vi "OverallControl.vi"(10 "Settings":T1={"Name of test"="", "Date"=timestamp(0 s since 1904-01-01), "Location"="", "Template"="", "Soundcard"="", "resolution"=0, "Sampling rate"=0, "Ch1 Gain "=0.0, "Ch2 Gain"=0.0, "Sample time (s)"=0.0, "Pre-trigger (s)"=0.0, "Hammer Threshold"=0.0, "Positions"=0, "Taps/Position"=0, "Set Names"="", "Freq resolution"=0.0, "Hammer cutoff"=0.0, "Mic cutoff"=0.0, "Double bounce "=0.0, "Hammer Cal"=0.0, "dB Offset"=0.0, "Accel Cal"=0.0, "Vibrometer Cal"=0.0, "Mic Cal"=0.0, "Output"=0, "Voltage Cal"=0.0, "Vibrometer Port"="", "Range"=0, "High Pass"=0, "Bandwidth"=0, "X Range"=[], "Y Range"=[], "dB Spread"=0.0, "Trigger"=0, "Ch_1"=0, "Ch_2"=0, "flip?"=FALSE, "60Hz"=FALSE, "Time offset"=0.0, "Piezo Cal"=1.0, "Default Notes"=""} {"Ch_2" min=1 step=1; "Ch_1" min=1 max=100 step=1; "Trigger" items=["Hammer (force)", "Self-tap", "Spacebar"]; "Bandwidth" items=["1 kHz"=1, "5 kHz"=5, "10 kHz"=10, "25 kHz"=25, "50 kHz"=50, "100 kHz"=100]; "High Pass" items=["Off", "13 Hz", "104 Hz"]; "Range" items=["10 mm/s"=1, "20 mm/s"=2, "50 mm/s"=5, "100 mm/s"=10, "200 mm/s"=20, "500 mm/s"=50, "1 m/s"=100, "2 m/s"=200]; "Output" items=["Accelerometer", "Speed (from acceleration)", "Microphone", "Vibrometer", "Piezo"]; "Voltage Cal" format="%#_13g"; "Ch2 Gain" format="%#_13g"; "Ch1 Gain" format="%#_13g"; "Double bounce" min=0.0; "Mic cutoff" min=0.0 format="%#_4g"; "Hammer cutoff" min=0.0 format="%#_4g"; "Freq resolution" min=0.0; "Pre-trigger (s)" format="%#_13g"; "Date" format="%<%H:%M\n%d/%m/%y>T"; "resolution" items=["16 bit"=16, "24 bit"=24, "32 bit"=32]; "Sampling rate" items=["22050 samp/s"=22050, "44100 samp/s"=44100, "48000 samp/s"=48000]}) -> (1 "Success?":bool, 3 "VISA Refnum out":refnum<visa-resource-name>)   [LabVIEW 2022 SP3]
uses:
  PreferencesControl.ctl
panel:
  out "Sent":string
  out "String Read":string
  # "Hz"
  # "dB"
  # "dB"
  # "sec"
  # "sec"
  # "mV/Pa"
  # "mV/m/s2"
  # "mV/mm/s"
  # "V/N"
  # "sec"
  # "sec"
  # "mV/N"
  # "a.u."
  # "a.u."
  # "sec"
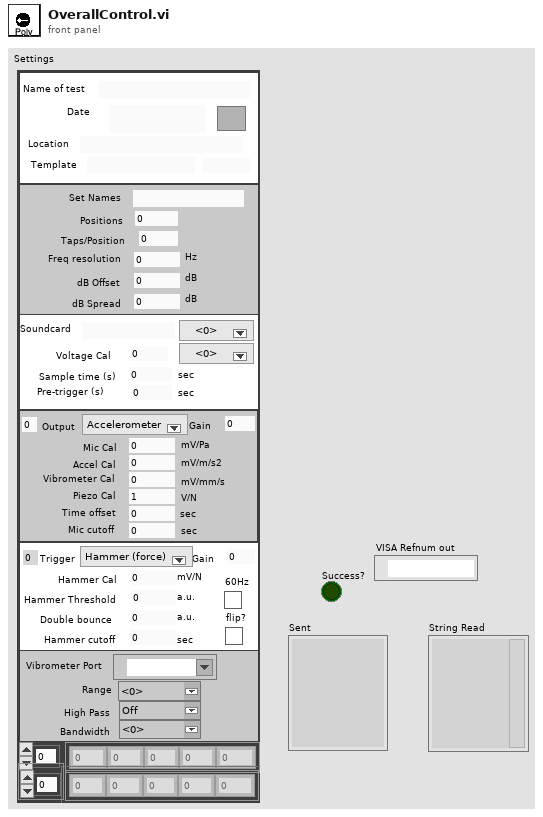
[diagram p1: front panel]
types:
  T1 = typedef "PreferencesControl.ctl" = cluster{"Name of test":string, "Date":timestamp, "Location":string, "Template":string, "Soundcard":string, "resolution":u16, "Sampling rate":u16, "Ch1 Gain ":dbl, "Ch2 Gain":dbl, "Sample time (s)":dbl, "Pre-trigger (s)":dbl, "Hammer Threshold":dbl, "Positions":i16, "Taps/Position":i16, "Set Names":string, "Freq resolution":dbl, "Hammer cutoff":dbl, "Mic cutoff":dbl, "Double bounce ":dbl, "Hammer Cal":dbl, "dB Offset":dbl, "Accel Cal":dbl, "Vibrometer Cal":dbl, "Mic Cal":dbl, "Output":u16, "Voltage Cal":dbl, "Vibrometer Port":refnum<visa-resource-name>, "Range":u16, "High Pass":u16, "Bandwidth":u16, "X Range":cluster{"Minimum":dbl, "Maximum":dbl, "Increment":dbl, "Minor Increment":dbl, "Start":dbl}[], "Y Range":cluster{"Minimum":dbl, "Maximum":dbl, "Increment":dbl, "Minor Increment":dbl, "Start":dbl}[], "dB Spread":dbl, "Trigger":u16, "Ch_1":u8, "Ch_2":u8, "flip?":bool, "60Hz":bool, "Time offset":dbl, "Piezo Cal":dbl, "Default Notes":string}
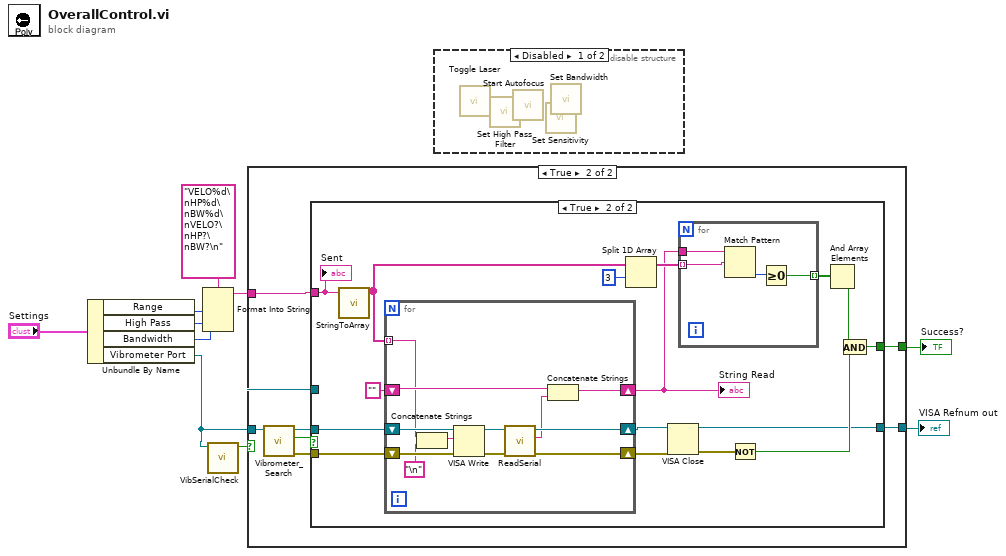
[diagram p0: block diagram]
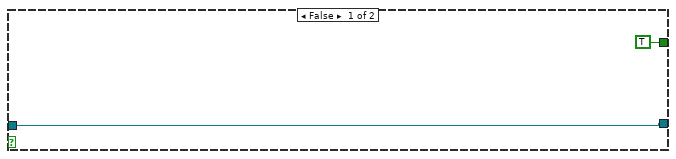
[diagram p3: hidden frame]
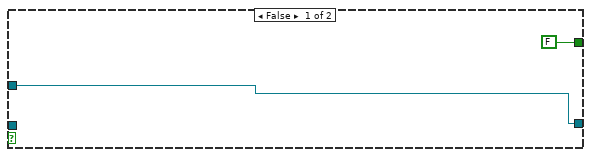
[diagram p4: hidden frame]
diagram:
  n1 = Unbundle By Name("Settings") -> ("Range"=w6:u16, "High Pass"=w7:u16, "Bandwidth"=w8:u16, "Vibrometer Port"=w2:refnum<visa-resource-name>)
  n2 = Format Into String(format string="VELO%d\nHP%d\nBW%d\nVELO?\nHP?\nBW?\n", w6, w7, w8) -> (resulting string=w5:string)  [unwired: 2 in, 1 out]
  n3 = call "VibSerialCheck.vi"("VISA Refnum in"=w2) -> ("Serial?"=w1:bool)  [unwired: 9 in, 1 out]
  n4 = case shown="True" w1 {
    tunnel: w5 -> [_ w19]
    tunnel: [TRUE w18] -> w4
    tunnel: [w12 w14] -> w3
    tunnel: w2 -> [w12 w13]
    frame False {
    }
    frame True {
      n5 = call "Vibrometer_Search.vi"("VISA Refnum in"=w13) -> ("error out"=w17:errorcluster, "Success?"=w15:bool, "VISA Refnum out"=w16:refnum<visa-resource-name>)  [unwired: 8 in]
      n6 = case shown="True" w15 {
        tunnel: w19 -> [_ w30]
        tunnel: [FALSE w26] -> w18
        tunnel: w17 -> [_ w24]
        tunnel: w16 -> [_ w23]
        tunnel: [w20 w22] -> w14
        tunnel: w13 -> [w20 _]
        frame False {
        }
        frame True {
          n7 = call "StringToArray.vi"("write buffer"=w30) -> ("Array"=w29:string[])  [unwired: 10 in]
          n8 = for {
            shift-right: [w52] -> w35
            shift-left: w24 -> [w50]
            shift-right: [w51] -> w22
            shift-left: w23 -> [w47]
            tunnel: w29 -> [w43] mode=indexing
            shift-right: [w44] -> w32
            shift-left: "" ("String Read") -> [w46]
            n9 = Concatenate Strings(w43, "\n" ("String Read")) -> (w41:string)
            n10 = VISA Write(VISA resource name=w47, write buffer=w41, error in (no error)=w50) -> (VISA resource name out=w49:refnum<visa-resource-name>, error out=w48:errorcluster)  [unwired: 1 out]
            n11 = call "ReadSerial.vi"("error in (no error)"=w48, "VISA Refnum in"=w49) -> ("error out"=w52:errorcluster, "String Read"=w45:string, "VISA Refnum out"=w51:refnum<visa-resource-name>)  [unwired: 7 in]
            n12 = Concatenate Strings(w46, w45) -> (w44:string)
          }
          "String Read" <- w32
          n13 = Split 1D Array(array=w29, index=3) -> (first subarray=w33:string[])  [unwired: 1 out]
          n14 = VISA Close(VISA resource name=w22, error in (no error)=w35) -> (error out=w27:errorcluster)
          n15 = for {
            tunnel: w33 -> [w39] mode=indexing
            tunnel: w32 -> [w40]
            tunnel: [w37] -> w31 mode=indexing
            n16 = Match Pattern(string=w40, regular expression=w39) -> (offset past match=w38:i32)  [unwired: 1 in, 3 out]
            n17 = Greater Or Equal To 0?(x=w38) -> (x >= 0?=w37:bool)
          }
          n18 = Not(x=w27) -> (.not. x?=w25:bool)
          n19 = And Array Elements(Boolean array=w31) -> (logical AND=w28:bool)
          n20 = And(x=w28, y=w25) -> (x .and. y?=w26:bool)
          "Sent" <- w30
        }
      }
    }
  }
  "Success?" <- w4
  "VISA Refnum out" <- w3
  n21 = disable-structure shown="Disabled" {
    frame Disabled {
      n22 = call "Toggle Laser.vi"() -> ()  [unwired: 10 in, 2 out]
      n23 = call "Set High Pass Filter.vi"() -> ()  [unwired: 10 in, 2 out]
      n24 = call "Start Autofocus.vi"() -> ()  [unwired: 10 in, 2 out]
      n25 = call "Set Sensitivity.vi"() -> ()  [unwired: 10 in, 2 out]
      n26 = call "Set Bandwidth.vi"() -> ()  [unwired: 10 in, 2 out]
    }
    frame Enabled {
    }
  }
